vi "Close.vi"(8 "error in (no error)":errorcluster, 11 "Class 1 in":refnum<class "csv.lvclass">) -> (0 "error out":errorcluster, 3 "Class 1 out":refnum<class "csv.lvclass">)   [LabVIEW 2021, in "Library.lvlib" / "csv.lvclass"]
uses:
  csv.lvclass
  csv.lvclass/csv.ctl
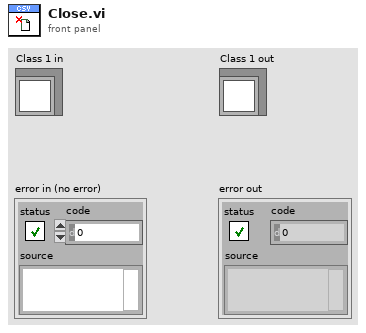
[diagram p1: front panel]
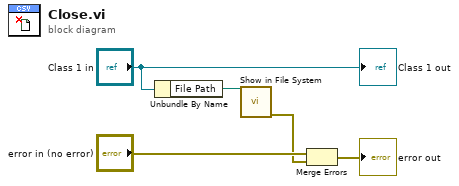
[diagram p0: block diagram]
diagram:
  n1 = Unbundle By Name("Class 1 in") -> ("File Path"=w3:path)
  n2 = call <vilib>:"Show in File System.vi"("file or directory path"=w3) -> ("error out"=w1:errorcluster)  [unwired: 10 in]
  n3 = Merge Errors("error in (no error)", w1) -> (→"error out":errorcluster)
  "Class 1 out" <- "Class 1 in"
